vi "_018.vi"() -> ()   [LabVIEW 2024]
panel:
  out "o/p":string
  in  "B":dbl
  in  "A":dbl
  out "Months No's":i32
  in  "Months":string
  out "Months":string
  in  "Months No's":dbl
  out "String":string
  in  "OK Button":bool
  in  "stop":bool
  # "Case Structures"
  # "It's equivalent to (if else & switch) in c || java  :"
  # "Months no.(Numeric) to Months (String) :"
  # "Months (String) to Months no.(Numeric) :"
  # "Logical Operator :"
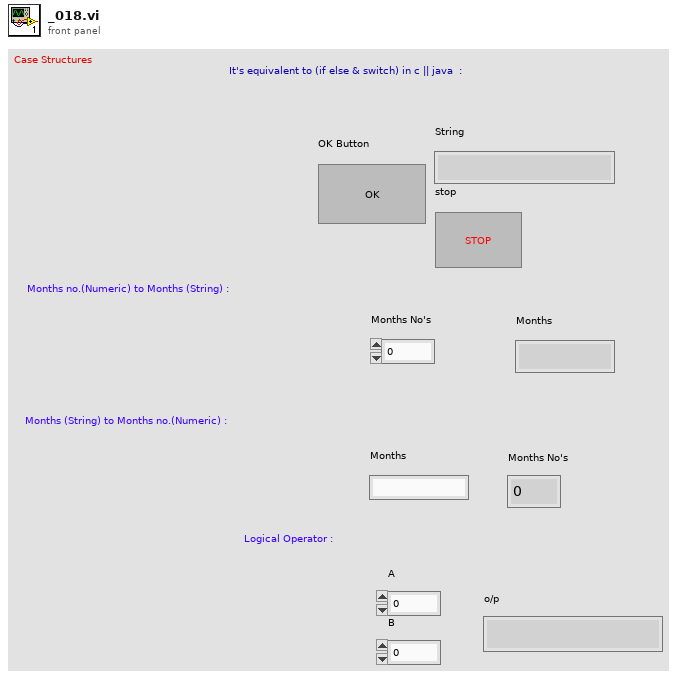
[diagram p1: front panel]
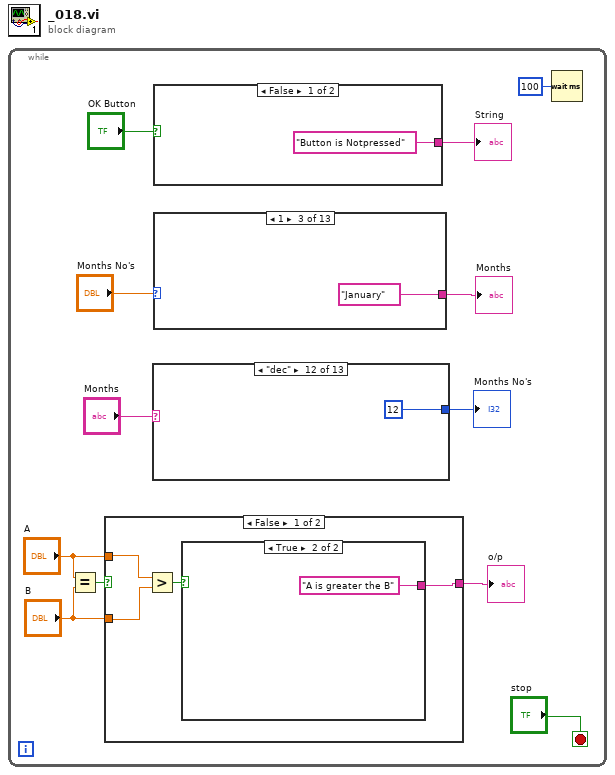
[diagram p0: block diagram]
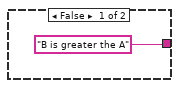
[diagram p2: hidden frame]
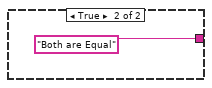
[diagram p3: hidden frame]
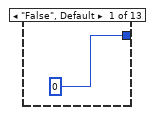
[diagram p4: hidden frame]
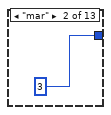
[diagram p5: hidden frame]
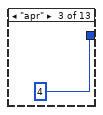
[diagram p6: hidden frame]
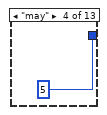
[diagram p7: hidden frame]
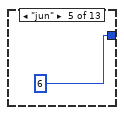
[diagram p8: hidden frame]
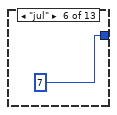
[diagram p9: hidden frame]
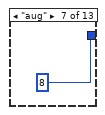
[diagram p10: hidden frame]
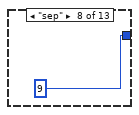
[diagram p11: hidden frame]
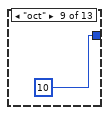
[diagram p12: hidden frame]
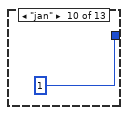
[diagram p13: hidden frame]
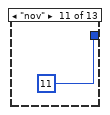
[diagram p14: hidden frame]
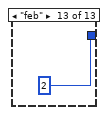
[diagram p15: hidden frame]
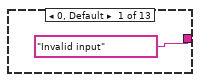
[diagram p16: hidden frame]
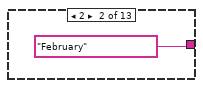
[diagram p17: hidden frame]
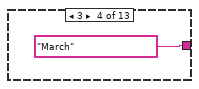
[diagram p18: hidden frame]
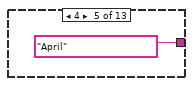
[diagram p19: hidden frame]
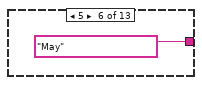
[diagram p20: hidden frame]
diagram:
  n1 = while {
    stop <- "stop" stop-if-true
    n2 = Equal?(x="A", y="B") -> (x = y?=w3:bool)
    n3 = case shown="False" w3 {
      tunnel: [w15 "Both are Equal"] -> w4
      tunnel: "A" -> [w14 _]
      tunnel: "B" -> [w13 _]
      frame False {
        n4 = Greater?(x=w14, y=w13) -> (0:w16:bool)
        n5 = case shown="True" w16 {
          tunnel: ["B is greater the A" "A is greater the B"] -> w15
          frame False {
          }
          frame True {
          }
        }
      }
      frame True {
      }
    }
    "o/p" <- w4
    n6 = case shown="\"dec\"" "Months" {
      tunnel: [0 3 4 5 6 7 8 9 10 1 11 12 2] -> w5
      frame "False", Default {
      }
      frame "mar" {
      }
      frame "apr" {
      }
      frame "may" {
      }
      frame "jun" {
      }
      frame "jul" {
      }
      frame "aug" {
      }
      frame "sep" {
      }
      frame "oct" {
      }
      frame "jan" {
      }
      frame "nov" {
      }
      frame "dec" {
      }
      frame "feb" {
      }
    }
    "Months No's" <- w5
    n7 = case shown="False" "OK Button" {
      tunnel: ["Button is Notpressed" "Button is pressed"] -> w9
      frame False {
      }
      frame True {
      }
    }
    "String" <- w9
    n8 = case shown="1" "Months No's" {
      tunnel: ["Invalid input" "February" "January" "March" "April" "May" "June" "July" "August" "September" "October" "November" "December"] -> w7
      frame 0, Default {
      }
      frame 2 {
      }
      frame 1 {
      }
      frame 3 {
      }
      frame 4 {
      }
      frame 5 {
      }
      frame 6 {
      }
      frame 7 {
      }
      frame 8 {
      }
      frame 9 {
      }
      frame 10 {
      }
      frame 11 {
      }
      frame 12 {
      }
    }
    "Months" <- w7
    n9 = Wait (ms)(milliseconds to wait=u32 100) -> ()  [unwired: 1 out]
  }
